vi "Humidity Control.vi"   [LabVIEW 2016]
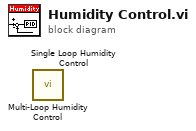
[diagram p0: block diagram]
diagram:
  n1 = call "Multi-Loop Humidity Control.vi"() -> ()  [unwired: 9 in, 3 out]
  n2 = call "Single Loop Humidity Control.vi"() -> ()  [unwired: 9 in, 3 out]
